vi "引用測試4.vi"() -> ()   [LabVIEW 2015]
uses:
  <vilib>/vision/Measure.llb/Edge Options.ctl
  <vilib>/vision/Measure.llb/Edge Polarity.ctl
  <vilib>/userdefined/High Color/IMAQdx.ctl
  <vilib>/vision/driver/NI_Vision_Acquisition_Software.lvlib
  <vilib>/vision/NI_Vision_Development_Module.lvlib
panel:
  in  "output cluster 2":cluster{"Data name":string, "Data":variant}
  out "output cluster":cluster{"Data name":string, "Data":variant}
  in  "Numeric":i32
  in  "ROI":T1=enum."Set Data"
  in  "動作":bool
  in  "重新開圖":bool
  out "Line Data":cluster{"X":sgl, "Y":sgl, "T":sgl}
  in  "開圖":bool
  in  "ShowData":bool
  in  "DieArea":i32=100 min=10
  in  "動作":enum16{"什麼也不做", "抓邊", "看灰階", "分析光源均勻度"}(ring)
  out "Mean":sgl format="%#.2f"
  out "Histogram":T2(graph)
  in  "取像":bool
  in  "Edge Options":T3={"Edge Polarity"=0, "Kernel Size"=3, "Width"=3, "Minimum Edge Strength"=10.0, "Interpolation Type"=enum."Bilinear Fixed", "Data Processing Method"=enum."Average"} {"Edge Polarity" items=["All Edges", "Rising Edges", "Falling Edges"]; "Minimum Edge Strength" format="%.2f"; "Width" step=2; "Kernel Size" step=2}
  out "error out":errorcluster
  out "Ellipse":T5 {"Minor Axis"."Point 2"."Y" format="%.2f"; "Minor Axis"."Point 2"."X" format="%.2f"; "Minor Axis"."Point 1"."Y" format="%.2f"; "Minor Axis"."Point 1"."X" format="%.2f"; "Major Axis"."Point 2"."Y" format="%.2f"; "Major Axis"."Point 2"."X" format="%.2f"; "Major Axis"."Point 1"."Y" format="%.2f"; "Major Axis"."Point 1"."X" format="%.2f"; "Center"."Y" format="%.2f"; "Center"."X" format="%.2f"}
  in  "圓":enum16{"Inner to Outer", "Outer to Inner"}(ring)
  out "Gradient Information":dbl[][](graph)
  in  "邊":T6(ring)
  in  "Process":T7(ring)
  in  "Gap":i32=10 min=1 max=300
  in  "stop":bool
  out "Image":T8(plugin-control)
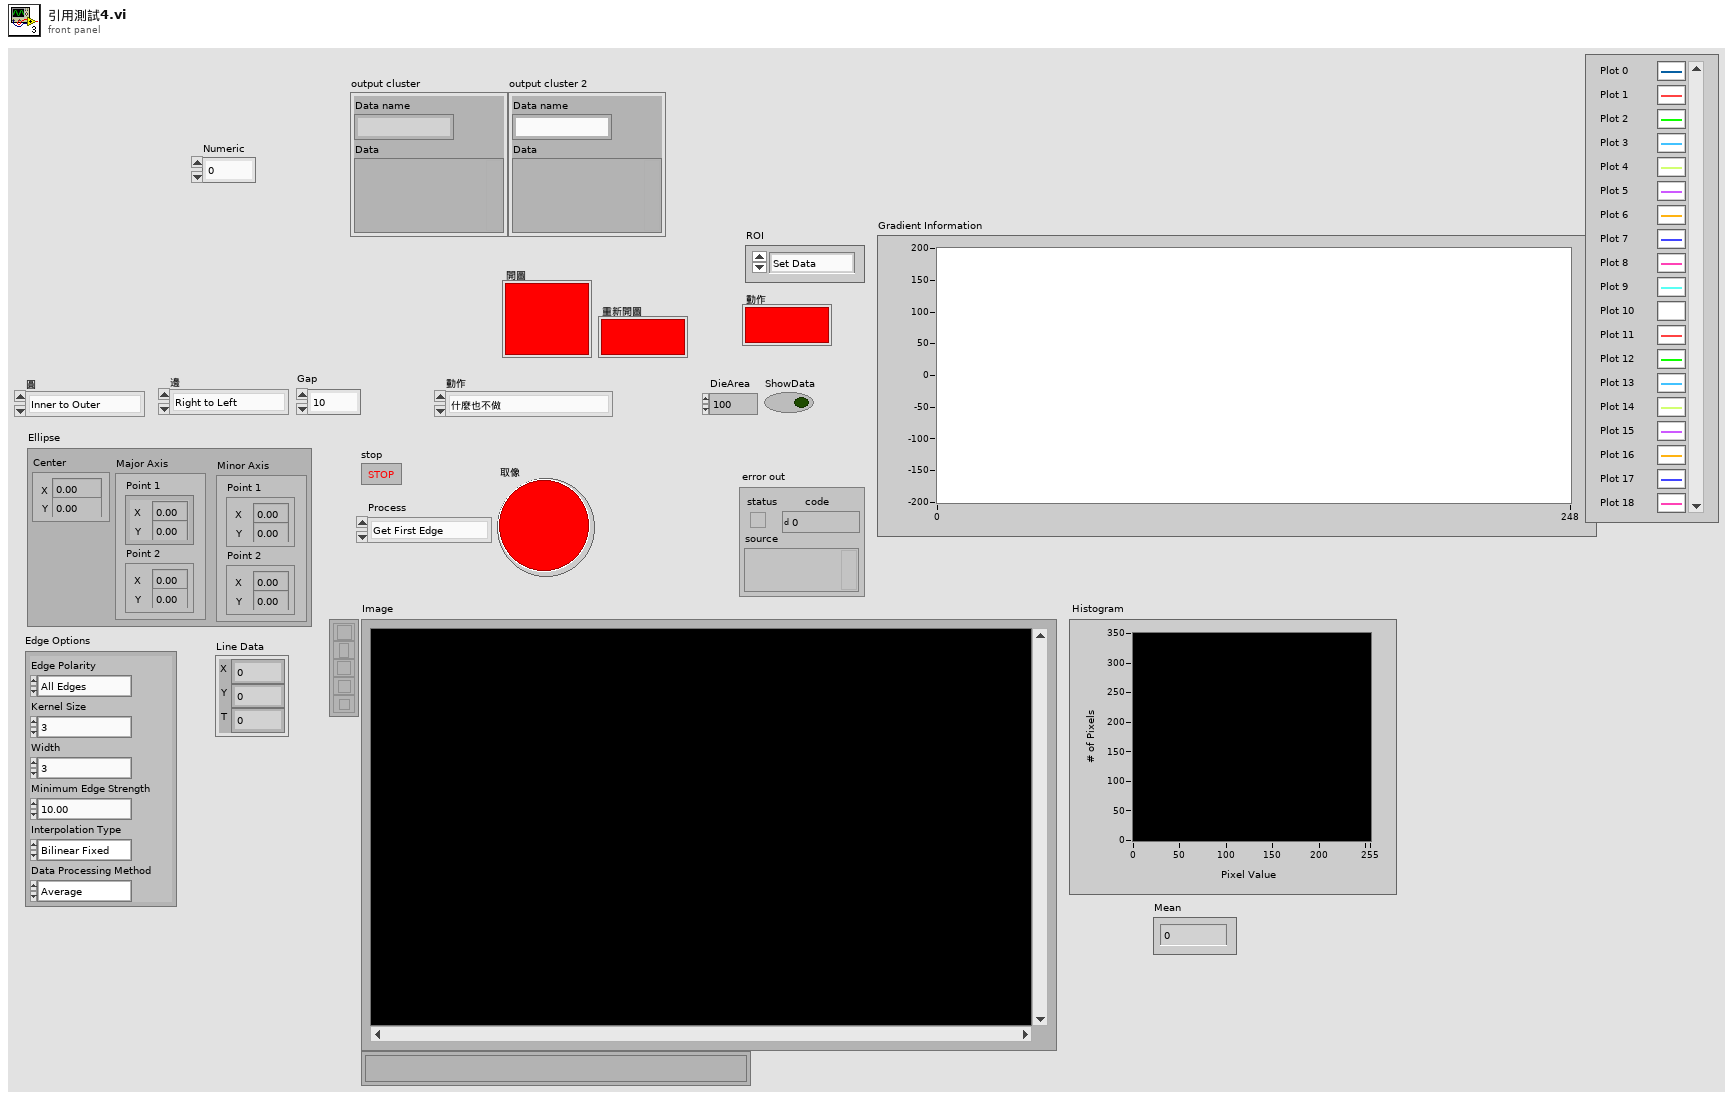
[diagram p1: front panel]
types:
  T1 = typedef "Action_Data.ctl" = enum16{"Initialize", "Get Data", "Set Data", "Delete Data", "Idle"}
  T2 = cluster{"Starting Value":sgl, "Incremental Value":sgl, "Histogram":u32[]}
  T3 = typedef "Edge Options.ctl" = cluster{"Edge Polarity":T4, "Kernel Size":u32, "Width":u32, "Minimum Edge Strength":sgl, "Interpolation Type":enum32{"Zero Order", "Bilinear", "Quadratic", "Cubic", "Bilinear Fixed"}, "Data Processing Method":enum32{"Average", "Median"}}
  T4 = typedef "Edge Polarity.ctl" = u32
  T5 = cluster{"Center":cluster{"X":sgl, "Y":sgl}, "Major Axis":cluster{"Point 1":cluster{"X":sgl, "Y":sgl}, "Point 2":cluster{"X":sgl, "Y":sgl}}, "Minor Axis":cluster{"Point 1":cluster{"X":sgl, "Y":sgl}, "Point 2":cluster{"X":sgl, "Y":sgl}}}
  T6 = enum16{"Right to Left", "Left  to Right", "Up to Down", "Down to Up"}
  T7 = enum16{"Get First Edge", "Get First + Last Edge", "Get All Edges", "Get Best Edge"}
  T8 = typedef "IMAQ Image.ctl" = refnum<image>
  T9 = typedef "IMAQ Rectangle" = cluster{"Left":i32, "Top":i32, "Right":i32, "Bottom":i32, "Rotation":dbl}
  T10 = typedef "IMAQdx.ctl" = refnum<k21>
  T11 = typedef "ROI Descriptor" = cluster{"Global Rectangle":i32[], "Contours":cluster{"ID":enum32{"External", "Internal"}, "Type":u32, "Coordinates":i32[]}[]}
  T12 = typedef "Image Type" = u32
  T13 = cluster{"Global Rectangle":i32[], "Contours":cluster{"Contour Type":u32, "ROI Type":u32, "Points":i32[]}[]}
  T14 = cluster{"Contour Type":u32, "ROI Type":u32, "Points":i32[]}[]
  T15 = cluster{"Contour Type":u32, "ROI Type":u32, "Points":i32[]}
  T16 = enum32{"Zero Order", "Bilinear", "Quadratic", "Cubic", "Bilinear Fixed"}
  T17 = cluster{"邊":enum16{"Right to Left", "Left  to Right", "Up to Down", "Down to Up"}, "動作":enum16{"什麼也不做", "抓邊", "看灰階", "分析光源均勻度"}, "圓":enum16{"Inner to Outer", "Outer to Inner"}, "Process":enum16{"Get First Edge", "Get First + Last Edge", "Get All Edges", "Get Best Edge"}, "ROI Type":u32, "Gap":i32, i32, i32, i32, i32, "Edge Polarity":T4, "Kernel Size":u32, "Width":u32, "Minimum Edge Strength":sgl, "Interpolation Type":enum32{"Zero Order", "Bilinear", "Quadratic", "Cubic", "Bilinear Fixed"}, "Data Processing Method":enum32{"Average", "Median"}, "DieArea":i32, "ShowData":bool}
  T18 = cluster{"邊":bool, "動作":bool, "圓":bool, "Process":bool, "ROI Type":bool, "Gap":bool, bool, bool, bool, bool, "Edge Polarity":bool, "Kernel Size":bool, "Width":bool, "Minimum Edge Strength":bool, "Interpolation Type":bool, "Data Processing Method":bool, "DieArea":bool, "ShowData":bool}
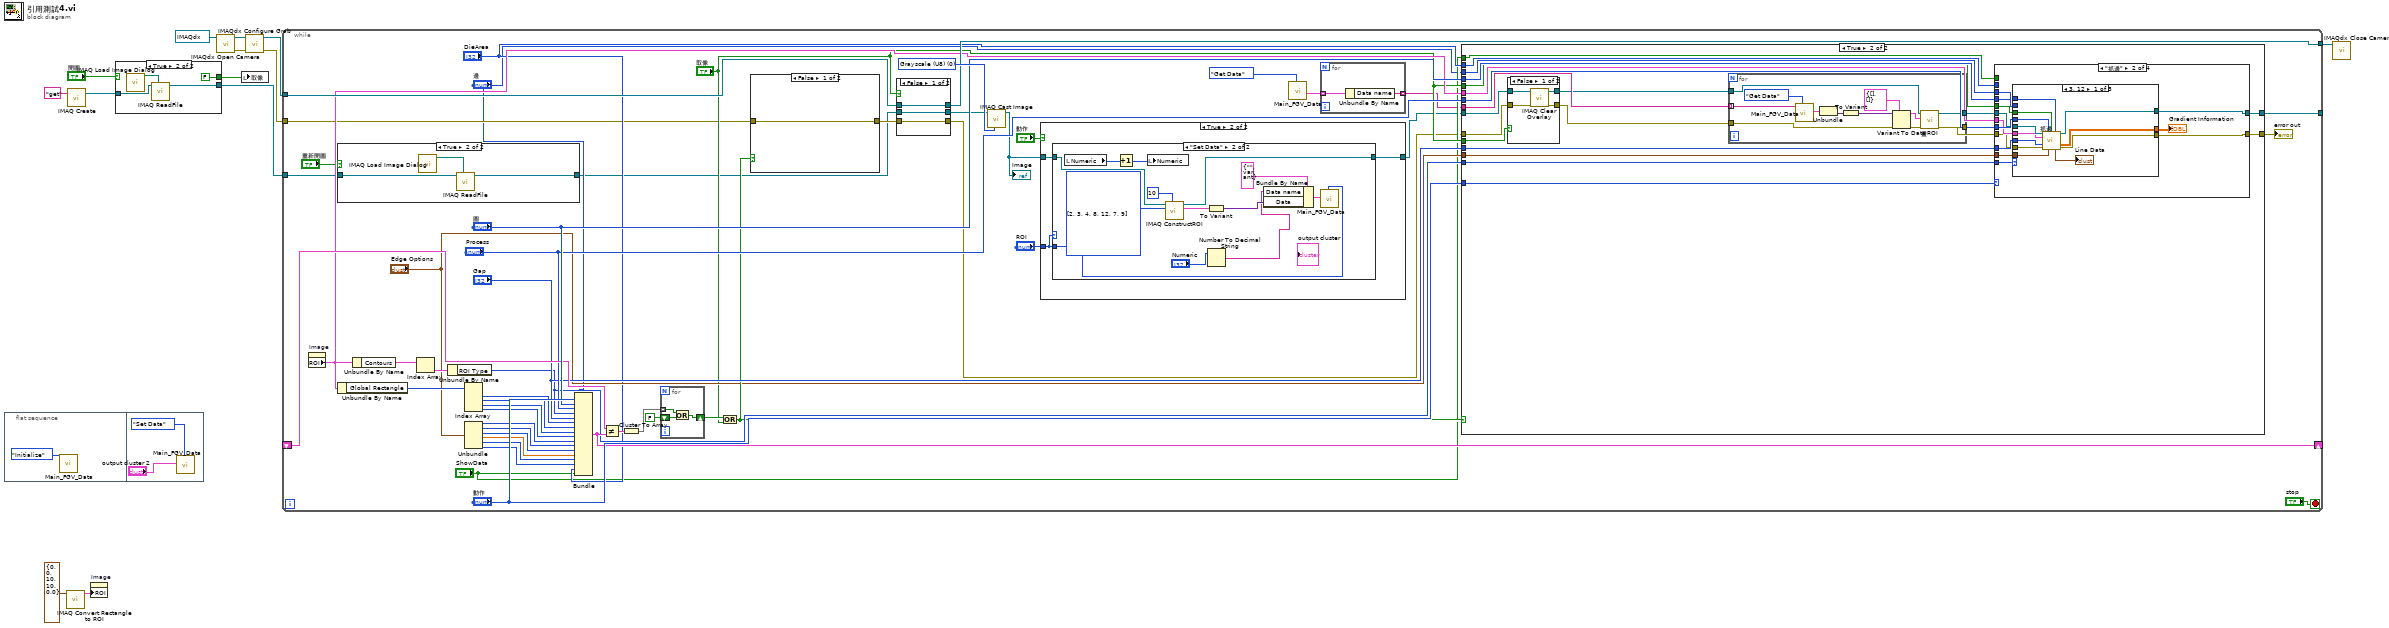
[diagram p0: block diagram]
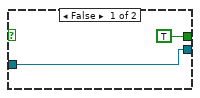
[diagram p2: hidden frame]
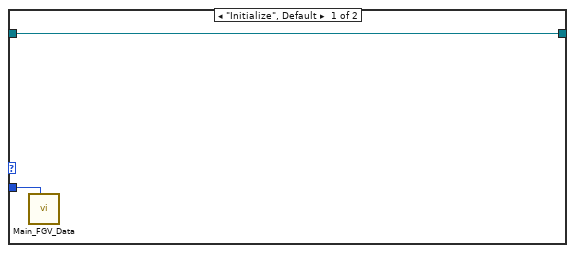
[diagram p4: hidden frame]
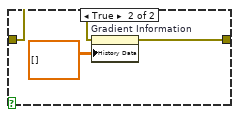
[diagram p6: hidden frame]
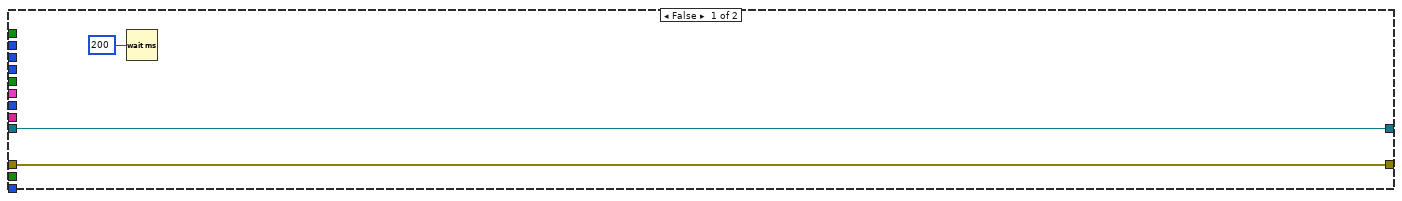
[diagram p7: hidden frame]
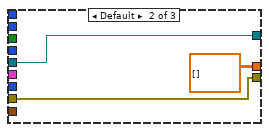
[diagram p10: hidden frame]
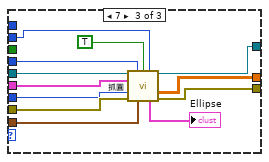
[diagram p11: hidden frame]
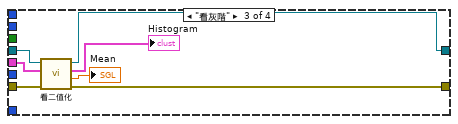
[diagram p12: hidden frame]
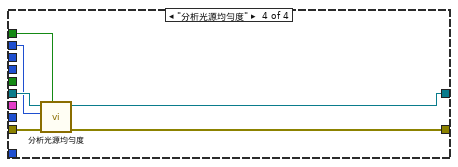
[diagram p13: hidden frame]
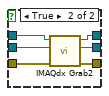
[diagram p14: hidden frame]
diagram:
  n1 = flat-sequence {
    frame #0 {
      n2 = call "Main_FGV_Data.vi"("Action_Data"=Action_Data."Initialize") -> ()  [unwired: 9 in, 2 out]
    }
    frame #1 {
      n3 = call "Main_FGV_Data.vi"("Action_Data"=Action_Data."Set Data", "Data In"="output cluster 2") -> ()  [unwired: 8 in, 2 out]
    }
  }
  n4 = call "IMAQ Convert Rectangle to ROI"("Rectangle"=T9 {"Left"=0, "Top"=0, "Right"=10, "Bottom"=10, "Rotation"=0.0}) -> ("ROI Descriptor"=w6:T11)  [unwired: 8 in, 1 out]
  n5 = call "IMAQ Create"("Image Name"="get") -> ("New Image"=w3:T8)  [unwired: 4 in, 1 out]
  n6 = property on="Image" class="ImageControl"("ROI"=w6) -> ()  [unwired: 2 in, 2 out]
  n7 = case shown="True" "開圖" {
    tunnel: [TRUE ("取像") FALSE ("取像")] -> w4
    tunnel: w3 -> [w17 w21]
    tunnel: [w17 w20] -> w2
    frame False {
    }
    frame True {
      n8 = call "IMAQ Load Image Dialog"() -> ("Path"=w19:path)  [unwired: 9 in, 2 out]
      n9 = call "IMAQ ReadFile"("File Path"=w19, "Image"=w21) -> ("Image Out"=w20:T8)  [unwired: 5 in, 4 out]
    }
  }
  n10 = call <vilib>:"IMAQdx Open Camera.vi"("Session In"=T10 "cam1") -> ("error out"=w8:errorcluster, "Session Out"=w9:T10)  [unwired: 9 in]
  n11 = local write "取像"(w4) -> ()
  n12 = call <vilib>:"IMAQdx Configure Grab.vi"("error in"=w8, "Session In"=w9) -> ("error out"=w1:errorcluster, "Session Out"=w12:T10)  [unwired: 8 in]
  n13 = while {
    tunnel: w12 -> [w73]
    tunnel: w2 -> [w32]
    tunnel: [w55] -> w11
    tunnel: [w69] -> _
    shift-right: [w64] -> _
    shift-left: _ -> [w63]
    tunnel: w1 -> [w36]
    stop <- "stop" stop-if-true
    w71 = T12 0 items=["Grayscale (U8)", "Grayscale (I16)", "Grayscale (SGL)", "Complex (CSG)", "RGB (U32)", "HSL (U32)", "RGB (U64)", "Grayscale (U16)"] ("Image Type")
    n14 = property on="Image" class="ImageControl"() -> ("ROI"=w53:T13)  [unwired: 2 in, 2 out]
    n15 = case shown="True" "重新開圖" {
      tunnel: w32 -> [w95 w96]
      tunnel: [w95 w97] -> w31
      frame False {
      }
      frame True {
        n16 = call "IMAQ Load Image Dialog"() -> ("Path"=w98:path)  [unwired: 9 in, 2 out]
        n17 = call "IMAQ ReadFile"("File Path"=w98, "Image"=w96) -> ("Image Out"=w97:T8)  [unwired: 5 in, 4 out]
      }
    }
    n18 = Unbundle By Name(w53) -> ("Global Rectangle"=w52:i32[])
    n19 = Unbundle By Name(w53) -> ("Contours"=w68:T14)
    n20 = Index Array(array=w68) -> (element=w67:T15)  [unwired: 1 in]
    n21 = Unbundle By Name(w67) -> ("ROI Type"=w57:u32)
    n22 = Index Array(array=w52) -> (element #1=w51:i32, element #2=w50:i32, element #3=w49:i32, element #4=w48:i32)  [unwired: 4 in]
    n23 = Unbundle("Edge Options") -> ("Edge Polarity"=w45:T4, "Kernel Size"=w44:u32, "Width"=w43:u32, "Minimum Edge Strength"=w42:sgl, "Interpolation Type"=w41:T16, "Data Processing Method"=w40:enum32{"Average", "Median"})
    n24 = Bundle("邊"="邊", "動作"="動作", "圓"="圓", "Process"="Process", "ROI Type"=w57, "Gap"="Gap", w51, w50, w49, w48, "Edge Polarity"=w45, "Kernel Size"=w44, "Width"=w43, "Minimum Edge Strength"=w42, "Interpolation Type"=w41, "Data Processing Method"=w40, "DieArea"="DieArea", "ShowData"="ShowData") -> (w64:T17)  [unwired: 1 in]
    n25 = Not Equal?(x=w63, y=w64) -> (x != y?=w56:T18)
    n26 = Cluster To Array(cluster=w56) -> (array=w62:bool[])
    n27 = for {
      tunnel: w62 -> [w105] mode=indexing
      shift-right: [w104] -> w60
      shift-left: FALSE -> [w103]
      n28 = Or(x=w105, y=w103) -> (x .or. y?=w104:bool)
    }
    n29 = Or(x=w60, y="取像") -> (x .or. y?=w47:bool)
    n30 = case shown="False" w47 {
      tunnel: [w99 w101] -> w70
      tunnel: w36 -> [w99 w100]
      frame False {
      }
      frame True {
        n31 = property on="Gradient Information" class="WFChart (strict)"(error in=w100, "History Data"=dbl[][] []) -> (error out=w101:errorcluster)  [unwired: 1 in, 1 out]
      }
    }
    n32 = case shown="False" "取像" {
      tunnel: w73 -> [w205 w211]
      tunnel: w31 -> [w204 w210]
      tunnel: [w205 w209] -> w55
      tunnel: [w204 w208] -> w54
      tunnel: w70 -> [w203 w207]
      tunnel: [w203 w206] -> w25
      frame False {
      }
      frame True {
        n33 = call <vilib>:"IMAQdx Grab2.vi"("error in"=w207, "Image In"=w210, "Session In"=w211) -> ("error out"=w206:errorcluster, "Image Out"=w208:T8, "Session Out"=w209:T10)  [unwired: 5 in, 1 out]
      }
    }
    n34 = call "IMAQ Cast Image"("Image Type"=w71, "Image Src"=w54) -> ("Image Dst Out"=w24:T8)  [unwired: 8 in, 1 out]
    "Image" <- w24
    n35 = case shown="True" "動作" {
      tunnel: w24 -> [w76 w79]
      tunnel: [w76 w78] -> w23
      tunnel: "ROI" -> [_ w77]
      frame False {
      }
      frame True {
        n36 = case shown="\"Set Data\"" w77 {
          tunnel: w79 -> [w81 w92]
          tunnel: [w81 w90] -> w78
          tunnel: w77 -> [w80 w84]
          frame "Initialize", Default {
            n37 = call "Main_FGV_Data.vi"("Action_Data"=w80) -> ()  [unwired: 9 in, 2 out]
          }
          frame "Set Data" {
            w94 = u32[] [2, 3, 4, 8, 12, 7, 9] items=["No Selection", "Point", "Line", "Rectangle", "Oval", "Polygon", "Freehand Region", "Annulus", "Zoom", "Pan", "Broken Line", "Freehand Line", "Rotated Rectangle"] ("Tools")
            n38 = local read "Numeric"() -> (w86:i32)
            n39 = Increment(x=w86) -> (x+1=w85:i32)
            n40 = local write "Numeric"(w85) -> ()
            n41 = call "IMAQ ConstructROI"("Window Number (-1...15)"=10, "Tools"=w94, "Image"=w92) -> ("ROI Descriptor Out"=w91:T11, "Image Out (duplicate)"=w90:T8)  [unwired: 5 in, 2 out]
            n42 = To Variant(anything=w91) -> (Variant=w89:variant)
            n43 = Number To Decimal String(number="Numeric") -> (decimal integer string=w82:string)  [unwired: 1 in]
            n44 = Bundle By Name(cluster=cluster{"Data name":string, "Data":variant} {"Data name"="", "Data"=variant} ("Data In"), "Data name"=w82, "Data"=w89) -> (w83:cluster{"Data name":string, "Data":variant})
            n45 = call "Main_FGV_Data.vi"("Action_Data"=w84, "Data In"=w83) -> ()  [unwired: 8 in, 2 out]
          }
        }
      }
    }
    n46 = call "Main_FGV_Data.vi"("Action_Data"=Action_Data."Get Data") -> ("Data Array out"=w29:cluster{"Data name":string, "Data":variant}[])  [unwired: 9 in, 1 out]
    n47 = for {
      tunnel: [w75] -> w26 mode=indexing
      tunnel: w29 -> [w74] mode=indexing
      n48 = Unbundle By Name(w74) -> ("Data name"=w75:string)
    }
    n49 = case shown="True" w47 {
      tunnel: "Gap" -> [_ w129]
      tunnel: w25 -> [w108 w114]
      tunnel: "Process" -> [_ w128]
      tunnel: w23 -> [w107 w119]
      tunnel: [w107 w127] -> w69
      tunnel: w53 -> [_ w126]
      tunnel: w57 -> [_ w125]
      tunnel: "Edge Options" -> [_ w124]
      tunnel: [w108 w123] -> w35
      tunnel: "動作" -> [_ w122]
      tunnel: "圓" -> [_ w121]
      tunnel: "取像" -> [_ w120]
      tunnel: "取像" -> [_ w118]
      tunnel: "DieArea" -> [_ w117]
      tunnel: "ShowData" -> [_ w116]
      tunnel: "邊" -> [_ w115]
      tunnel: w26 -> [_ w112]
      frame False {
        n50 = Wait (ms)(milliseconds to wait=u32 200) -> ()  [unwired: 1 out]
      }
      frame True {
        n51 = case shown="False" w120 {
          tunnel: w119 -> [w144 w147]
          tunnel: [w145 w147] -> w110
          tunnel: w114 -> [w143 w146]
          tunnel: [w142 w146] -> w111
          frame False {
            n52 = call "IMAQ Clear Overlay"("error in (no error)"=w143, "Image"=w144) -> ("error out"=w142:errorcluster, "Image Out"=w145:T8)  [unwired: 8 in]
          }
          frame True {
          }
        }
        n53 = for {
          tunnel: w110 -> [w141]
          tunnel: [w140] -> w109
          tunnel: w111 -> [w131]
          tunnel: [w130] -> w113
          tunnel: w112 -> [w132] mode=indexing
          n54 = call "Main_FGV_Data.vi"("Action_Data"=Action_Data."Get Data", "Data name"=w132) -> ("Data  Out"=w138:cluster{"Data name":string, "Data":variant})  [unwired: 8 in, 1 out]
          n55 = Unbundle(w138) -> ("Data"=w137:variant)  [unwired: 1 out]
          n56 = To Variant(anything=w137) -> (Variant=w136:variant)
          n57 = Variant To Data(error in=w131, type=T11 {"Global Rectangle"=[], "Contours"=[]} ("ROI Descriptor"), Variant=w136) -> (data=w134:T11, error out=w133:errorcluster)
          n58 = call "畫ROI.vi"("error in (no error)"=w133, "ROI In"=w134, "Image In"=w141) -> ("error out"=w130:errorcluster, "Image"=w140:T8)  [unwired: 6 in, 1 out]
        }
        n59 = case shown="\"抓邊\"" w122 {
          tunnel: w129 -> [_ w162 _ _]
          tunnel: w113 -> [w148 w150 w193 w198]
          tunnel: w121 -> [_ w161 _ _]
          tunnel: w128 -> [_ w160 _ _]
          tunnel: w109 -> [w149 w159 w195 w200]
          tunnel: [w149 w158 w196 w201] -> w127
          tunnel: w126 -> [_ w157 w194 _]
          tunnel: w125 -> [_ w156 _ _]
          tunnel: w124 -> [_ w155 _ _]
          tunnel: [w148 w153 w190 w202] -> w123
          tunnel: w118 -> [_ w152 _ _]
          tunnel: w117 -> [_ _ _ w199]
          tunnel: w116 -> [_ _ _ w197]
          tunnel: w115 -> [_ w151 _ _]
          frame "什麼也不做", Default {
          }
          frame "抓邊" {
            n60 = case shown="3, 12" w156 {
              tunnel: w157 -> [w173 _ w183]
              tunnel: w162 -> [w172 _ w184]
              tunnel: w150 -> [w171 w175 w185]
              tunnel: w161 -> [_ _ w180]
              tunnel: w160 -> [w166 _ w181]
              tunnel: [w169 dbl[][] [] ("Gradient Information") w188] -> w154
              tunnel: w159 -> [w174 w177 w182]
              tunnel: [w168 w177 w189] -> w158
              tunnel: [w170 w175 w178] -> w153
              tunnel: w155 -> [w167 _ w186]
              tunnel: w152 -> [w165 _ _]
              tunnel: w151 -> [w163 _ _]
              frame 3, 12 {
                n61 = call "抓邊.vi"("Image In"=w174, "Process"=w166, "Optimized Mode"=w165, "Direction"=w163, "ROI"=w173, "Gap"=w172, "error In"=w171, "Edge Options"=w167) -> ("Image Out"=w168:T8, "Gradient Information"=w169:dbl[][], "Line Data"=→"Line Data":cluster{"X":sgl, "Y":sgl, "T":sgl}, "error out"=w170:errorcluster)  [unwired: 3 in, 1 out]
              }
              frame Default {
              }
              frame 7 {
                n62 = call "抓圓.vi"("Image In"=w182, "Process"=w181, "Optimized Mode"=TRUE, "Direction"=w180, "ROI"=w183, "Gap"=w184, "error In"=w185, "Edge Options"=w186) -> ("Imag e Out"=w189:T8, "Gradient Information"=w188:dbl[][], "Ellipse"=→"Ellipse":T5, "error out"=w178:errorcluster)  [unwired: 3 in, 1 out]
              }
            }
            "Gradient Information" <- w154
          }
          frame "看灰階" {
            n63 = call "看二值化.vi"("error in (no error)"=w193, "ROI Descriptor"=w194, "Image In"=w195) -> ("error out"=w190:errorcluster, "Mean"=→"Mean":sgl, "Histogram"=→"Histogram":T2, "Image Out"=w196:T8)  [unwired: 4 in, 1 out]
          }
          frame "分析光源均勻度" {
            n64 = call "分析光源均勻度.vi"("ShowData"=w197, "error in (no error)"=w198, "DieArea"=w199, "Image In"=w200) -> ("error out"=w202:errorcluster, "Image"=w201:T8)  [unwired: 6 in]
          }
        }
      }
    }
    "error out" <- w35
  }
  n65 = call <vilib>:"IMAQdx Close Camera.vi"("Session In"=w11) -> ()  [unwired: 10 in, 1 out]
